vi "Write right terminal.vi"(5 "right terminal":refnum<class "Terminal.lvclass">, 9 "FlatSequenceInnerTunnel in":refnum<class "FlatSequenceInnerTunnel.lvclass">) -> (3 "FlatSequenceInnerTunnel out":refnum<class "FlatSequenceInnerTunnel.lvclass">)   [LabVIEW 2014, in "FlatSequenceInnerTunnel.lvclass"]
uses:
  FlatSequenceInnerTunnel.lvclass
  Terminal/Terminal.lvclass
  FlatSequenceInnerTunnel.lvclass/FlatSequenceInnerTunnel.ctl
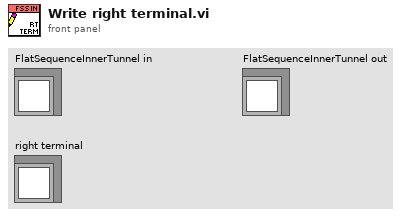
[diagram p1: front panel]
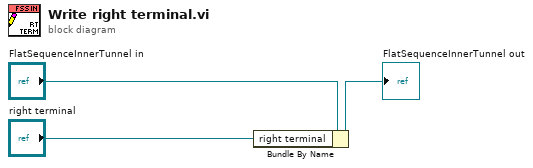
[diagram p0: block diagram]
diagram:
  n1 = Bundle By Name(cluster="FlatSequenceInnerTunnel in", "right terminal"="right terminal") -> (→"FlatSequenceInnerTunnel out":refnum<class "FlatSequenceInnerTunnel.lvclass">)
